vi "Drive Teleop.vi"(9 "POVs":i16[](array[numeric]), 10 "Boolean Array":bool[](array[boolean]), 11 "Axes":dbl[](array[numeric])) -> ()   [LabVIEW 2020]
uses:
  ADIS16470/Typedef/ADIS16470 Status.ctl
  ADIS16470/Typedef/ADIS16470 Data.ctl
  Scaling Types.ctl
  Axes.ctl
  Swerve Mode.ctl
  Buttons.ctl
  <vilib>/Rock Robotics/WPI/Joystick/XBox Buttons Indexer.ctl
  7d80139a-4be2-4268-81d7-0f551d61f1ba.vi
  e6f839d3-980b-4d83-88b4-2e0ae51acaef.vi
  <vilib>/Rock Robotics/Network Tables/NT Write Number.vi
  Drive/Implementation/Infrastructure/Drive Command Helper.vi
panel:
  in  "Rotation Scaling Type":T1
  in  "Translation Scaling Type":T1
  out "ADIS16470 Value":T2
  out "ADIS16470 Status":T3
  in  "Calibrate IMU":bool
  in  "Reset IMU":bool
  in  "Deadband":dbl=0.1
  in  "Disable Rotation":bool
  in  "Disable Y":bool
  in  "Disable X":bool
  in  "omega_max":dbl=180.0
  in  "v_max":dbl=10.0
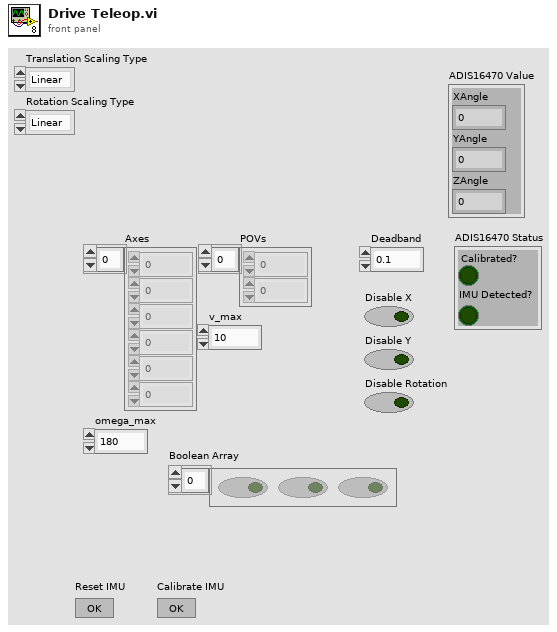
[diagram p1: front panel]
types:
  T1 = typedef "Scaling Types.ctl" = enum16{"Linear", "Square", "Cube", "RSVP5"}
  T2 = typedef "ADIS16470 Data.ctl" = cluster{"XAngle":dbl, "YAngle":dbl, "ZAngle":dbl}
  T3 = typedef "ADIS16470 Status.ctl" = cluster{"Calibrated?":bool, "IMU Detected?":bool}
  T4 = typedef "XBox Buttons Indexer.ctl" = enum16{"A", "B", "X", "Y", "Left Bumper", "Right Bumper", "Back", "Start", "Left Joystick", "Right Joystick"}
  T5 = typedef "Buttons.ctl" = enum16{"A", "B", "X", "Y", "LB", "RB", "menu", "start", "left stick", "right stick"}
  T6 = typedef "Swerve Mode.ctl" = enum16{"Robot Centric", "Field Centric"}
  T7 = typedef "Axes.ctl" = enum16{"LX", "LY", "LT", "RT", "RX", "RY"}
  T8 = typedef "ADIS16470 Device Reference.ctl" = cluster{"DevStatus":errorcluster, "Hardware Config":T9, "Calibration Complete":refnum<notifier>, "Status Reference":refnum<data-value>, "Position Reference":refnum<data-value>, "Velocity Reference":refnum<data-value>, "Sychronous Process VI":T13, "Cmd FIFO":refnum<k33>, "Source":T14, "Data FIFO":refnum<k33>, "Calibration Time (ms)":u32}
  T9 = typedef "ADIS16470 Hardware Configuration.ctl" = cluster{"SPI Clock Rate (Hz)":dbl, "IMU SPI Mode (3)":T10, "IMU Reset Pin":T11, "IMU SPI Bus":T12, "IMU Data Ready Pin":T11, "Stall Config":cluster{"Pow2BytesPerRead":u8, "StallTicks":u16, "CsToSclkTicks":u8}}
  T10 = typedef "WPI_SPIMode.ctl" = enum16{"Mode 0 (Clk Idle Low,Sample on Leading)", "Mode 1 (Clk Idle Low,Sample on Trailing)", "Mode 2 (Clk Idle High,Sample on Leading)", "Mode 3 (Clk Idle High,Sample on Trailing)"}
  T11 = typedef "FPGA_DIOChannel.ctl" = enum8{"DIO 0", "DIO 1", "DIO 2", "DIO 3", "DIO 4", "DIO 5", "DIO 6", "DIO 7", "DIO 8", "DIO 9", "DIO MXP 0", "DIO MXP 1", "DIO MXP 2", "DIO MXP 3", "DIO MXP 4", "DIO MXP 5", "DIO MXP 6", "DIO MXP 7", "DIO MXP 8", "DIO MXP 9", "DIO MXP 10", "DIO MXP 11", "DIO MXP 12", "DIO MXP 13", "DIO MXP 14", "DIO MXP 15", "SPI Port CS1", "SPI Port CS2", "SPI Port CS3", "SPI Port MISO", "SPI Port MOSI", "Invalid"}
  T12 = typedef "spi_bus.ctl" = enum16{"SPI On-Board, CS0", "SPI On-Board, CS1", "SPI On-Board, CS2", "SPI On-Board, CS3", "SPI MXP", "Invalid"}
  T13 = typedef "ADIS16470 Process.ctl" = refnum<vi>
  T14 = typedef "FPGA_CounterEncoderSourceConvertionLVSourceType.ctl" = cluster{"DevStatus":errorcluster, "AnalogTriggerMode?":bool, "DigitalMode":cluster{"DIO Channel":T15}, "AnalogTriggerMode":cluster{"AnalogTriggerIndex":T16, "OutputType":T17}}
  T15 = typedef "FPGA_DIODigitalSourceChannel.ctl" = enum8{"DIO 0", "DIO 1", "DIO 2", "DIO 3", "DIO 4", "DIO 5", "DIO 6", "DIO 7", "DIO 8", "DIO 9", "DIO MXP 0", "DIO MXP 1", "DIO MXP 2", "DIO MXP 3", "DIO MXP 4", "DIO MXP 5", "DIO MXP 6", "DIO MXP 7", "DIO MXP 8", "DIO MXP 9", "DIO MXP 10", "DIO MXP 11", "DIO MXP 12", "DIO MXP 13", "DIO MXP 14", "DIO MXP 15", "SPI Port CS1", "SPI Port CS2", "SPI Port CS3", "SPI Port MISO", "SPI Port MOSI", "Disabled"}
  T16 = typedef "FPGA_AnalogTriggerIndex.ctl" = enum8{"Trig 0", "Trig 1", "Trig 2", "Trig 3", "Trig 4", "Trig 5", "Trig 6", "Trig 7", "Invalid"}
  T17 = typedef "FPGA_AnalogTriggerOutType.ctl" = enum16{"InWindow", "TriggerState", "Rising", "Falling"}
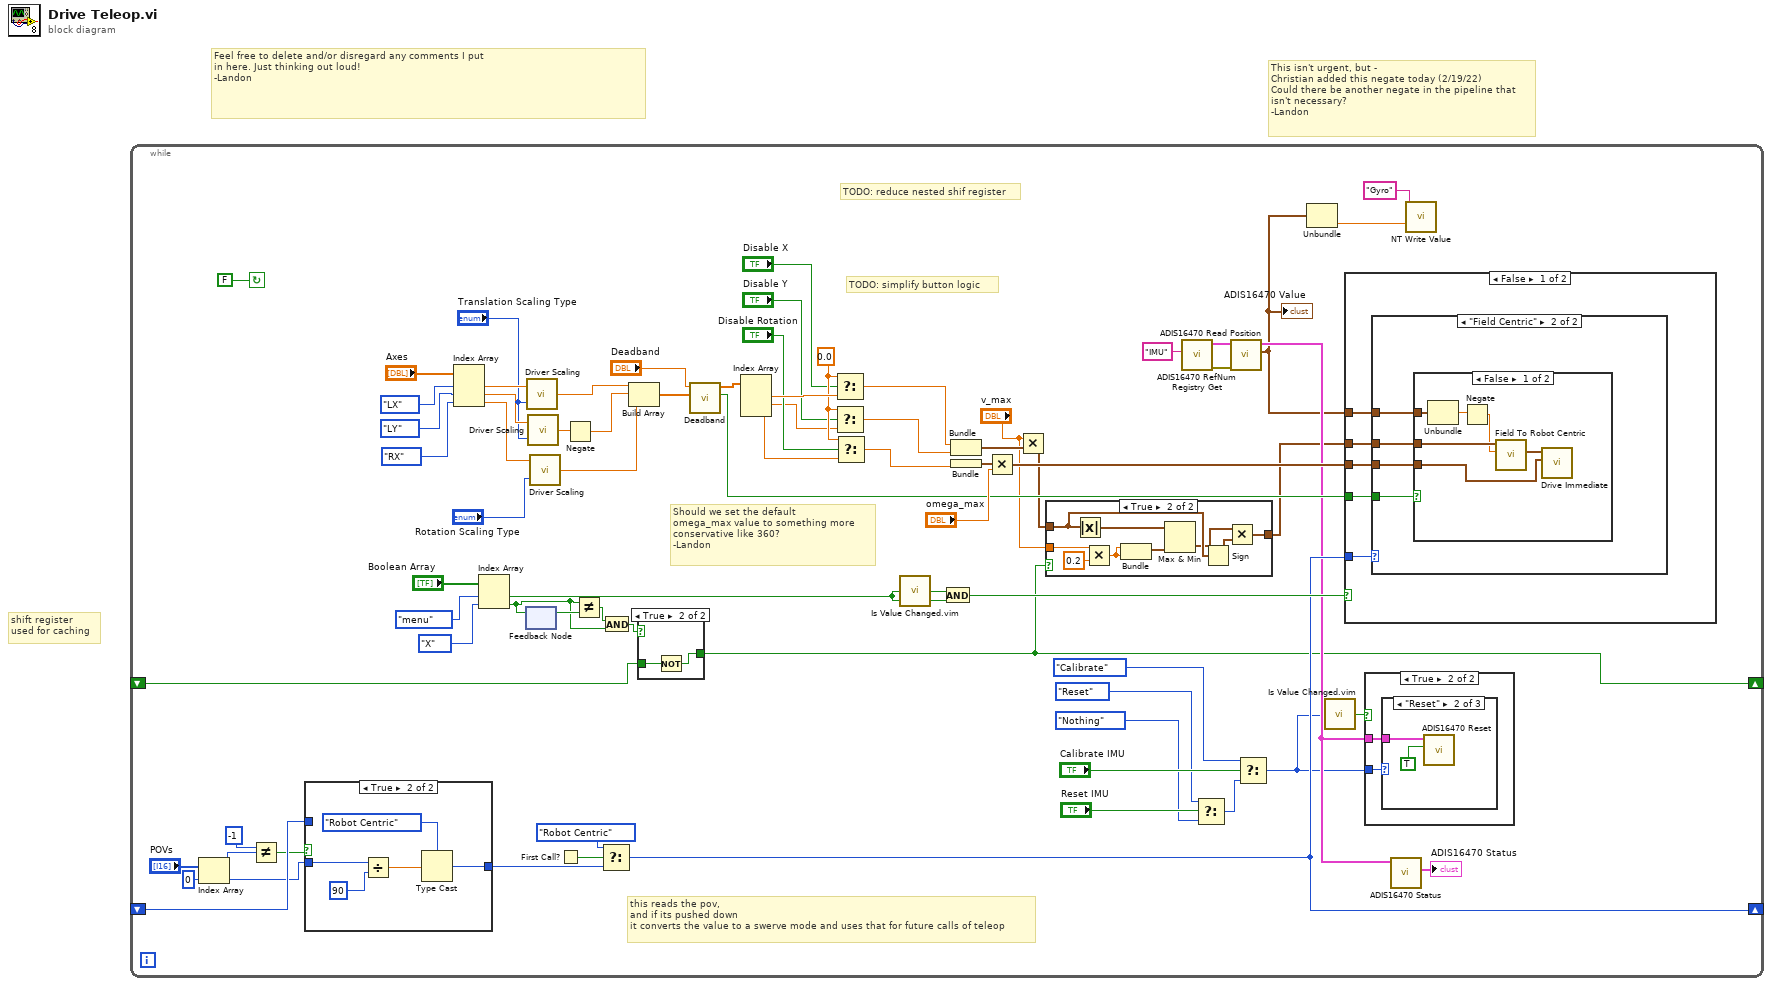
[diagram p0: block diagram]
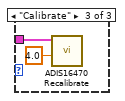
[diagram p6: hidden frame]
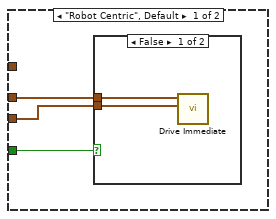
[diagram p7: hidden frame]
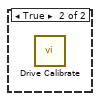
[diagram p10: hidden frame]
diagram:
  # "Feel free to delete and/or disregard any comments I put\nin here. Just thinking out loud!\n-Landon"
  # "This isn't urgent, but -\nChristian added this negate today (2/19/22)\nCould there be another negate in the pipeline that\nisn't necessary?\n-Landon"
  # "shift register\nused for caching"
  n1 = while {
    shift-right: [w39] -> _
    shift-left: _ -> [w65]
    shift-right: [w10] -> _
    shift-left: _ -> [w11]
    stop <- FALSE continue-if-true
    w59 = 0.0 ("f")
    # "Should we set the default\nomega_max value to something more\nconservative like 360?\n-Landon"
    # "TODO: simplify button logic"
    # "TODO: reduce nested shif register"
    # "this reads the pov,\nand if its pushed down\nit converts the value to a swerve mode and uses that for future calls of teleop"
    n2 = Index Array(array="POVs", index=0) -> (element=w46:i16)
    n3 = Not Equal?(x=-1, y=w46) -> (x != y?=w47:bool)
    n4 = case shown="True" w47 {
      tunnel: w46 -> [_ w118]
      tunnel: [w113 w114] -> w66
      tunnel: w65 -> [w113 _]
      frame False {
      }
      frame True {
        n5 = Divide(x=w118, y=90) -> (x/y=w115:dbl)
        n6 = Type Cast(type=Swerve_Mode."Robot Centric" ("Swerve Mode"), x=w115) -> (*(type *) &x=w114:T6)
      }
    }
    n7 = Index Array(array="Axes", index #1=Axes."LX" ("Axes"), index #2=Axes."LY" ("Axes"), index #3=Axes."RX" ("Axes")) -> (element #1=w24:dbl, element #2=w23:dbl, element #3=w22:dbl)
    n8 = Index Array(array="Boolean Array", index #1=Buttons."menu" ("Button"), index #2=XBox_Buttons_Indexer."X" ("XBox Buttons")) -> (element #1=w13:bool, element #2=w5:bool)
    n9 = feedback-in #1(w5) -> ()
    n10 = feedback #1() -> (w12:bool)  [unwired: 1 in]
    n11 = call "Driver Scaling.vi"("Scaling Type"="Translation Scaling Type", "x"=w24) -> ("y"=w17:dbl)
    n12 = call "Driver Scaling.vi"("Scaling Type"="Translation Scaling Type", "x"=w23) -> ("y"=w19:dbl)
    n13 = call "Driver Scaling.vi"("Scaling Type"="Rotation Scaling Type", "x"=w22) -> ("y"=w16:dbl)
    n14 = First Call?() -> (First Call?: T/F=w68:bool)
    n15 = Negate(x=w19) -> (-x=w18:dbl)
    n16 = Not Equal?(x=w5, y=w12) -> (x != y?=w6:bool)
    n17 = Select(t=Swerve_Mode."Robot Centric" ("Swerve Mode"), s=w68, f=w66) -> (s? t:f=w39:T6)
    n18 = And(x=w6, y=w5) -> (x .and. y?=w4:bool)
    n19 = Build Array(w17, w18, w16) -> (w15:dbl[])
    n20 = case shown="True" w4 {
      tunnel: w11 -> [w84 w86]
      tunnel: [w84 w85] -> w10
      frame False {
      }
      frame True {
        n21 = Not(x=w86) -> (.not. x?=w85:bool)
      }
    }
    n22 = call "Deadband.vi"("Inputs"=w15, "Deadband"="Deadband") -> ("Is Zero?"=w40:bool, "Ouptuts"=w41:dbl[])  [unwired: 8 in]
    n23 = Index Array(array=w41) -> (element #1=w61:dbl, element #2=w51:dbl, element #3=w60:dbl)  [unwired: 3 in]
    n24 = Select(t=w59, s="Disable X", f=w61) -> (s? t:f=w55:dbl)
    n25 = Select(t=w59, s="Disable Y", f=w51) -> (s? t:f=w54:dbl)
    n26 = Select(t=w59, s="Disable Rotation", f=w60) -> (s? t:f=w53:dbl)
    n27 = call "Is Value Changed.vim"("value"=w13) -> ("changed or first call?"=w43:bool)
    n28 = And(x=w43, y=w13) -> (x .and. y?=w45:bool)
    n29 = Bundle("upper limit"=w55, "upper limit"=w54) -> (w52:cluster{"upper limit":dbl, "upper limit":dbl})  [unwired: 1 in]
    n30 = Bundle("upper limit"=w53) -> (w64:cluster{"upper limit":dbl})  [unwired: 1 in]
    n31 = Multiply(x=w64, y="omega_max") -> (x*y=w62:cluster{"upper limit":dbl})
    n32 = Multiply(x="v_max", y=w52) -> (x*y=w9:cluster{"upper limit":dbl, "upper limit":dbl})
    n33 = case shown="True" w10 {
      tunnel: w9 -> [w74 w78]
      tunnel: "v_max" -> [_ w81]
      tunnel: [w74 w76] -> w7
      frame False {
      }
      frame True {
        n34 = Absolute Value(x=w78) -> (abs(x)=w83:cluster{"upper limit":dbl, "upper limit":dbl})
        n35 = Multiply(x=w81, y=0.2) -> (x*y=w79:dbl)
        n36 = Bundle(w79, w79) -> (w82:cluster{dbl, dbl})  [unwired: 1 in]
        n37 = Max & Min(x=w83, y=w82) -> (min(x,y)=w75:cluster{dbl, dbl})  [unwired: 1 out]
        n38 = Sign(1:w78) -> (0:w77:cluster{"upper limit":dbl, "upper limit":dbl})
        n39 = Multiply(x=w75, y=w77) -> (x*y=w76:cluster{dbl, dbl})
      }
    }
    n40 = call "ADIS16470 RefNum Registry Get.vi"("refnum name"="IMU") -> ("error out"=w38:errorcluster, "ADIS16470DevRef out"=w37:T8)  [unwired: 9 in]
    n41 = Select(t=enum16{"Nothing", "Calibrate", "Reset"}."Reset", s="Reset IMU", f=enum16{"Nothing", "Calibrate", "Reset"}."Nothing") -> (s? t:f=w31:enum16{"Nothing", "Calibrate", "Reset"})
    n42 = call "ADIS16470 Read Position.vi"("error in (no error)"=w38, "ADIS16470DevRef"=w37) -> ("ADIS16470 Value"=w3:T2, "ADIS16470DevRef"=w30:T8)  [unwired: 6 in, 2 out]
    "ADIS16470 Value" <- w3
    n43 = Select(t=enum16{"Nothing", "Calibrate", "Reset"}."Calibrate", s="Calibrate IMU", f=w31) -> (s? t:f=w28:enum16{"Nothing", "Calibrate", "Reset"})
    n44 = Unbundle(w3) -> ("ZAngle"=w1:dbl)  [unwired: 2 out]
    n45 = call "Is Value Changed.vim"("value"=w28) -> ("changed or first call?"=w27:bool)
    n46 = case shown="False" w45 {
      tunnel: w62 -> [w97 _]
      tunnel: w7 -> [w96 _]
      tunnel: w40 -> [w95 _]
      tunnel: w39 -> [w94 _]
      tunnel: w3 -> [w93 _]
      frame False {
        n47 = case shown="\"Field Centric\"" w94 {
          tunnel: w97 -> [w100 w105]
          tunnel: w96 -> [w99 w106]
          tunnel: w95 -> [w98 w103]
          tunnel: w93 -> [_ w104]
          frame "Robot Centric", Default {
            n48 = case shown="False" w98 {
              tunnel: w100 -> [w101 _]
              tunnel: w99 -> [w102 _]
              frame False {
                n49 = call "Drive Immediate.vi"("Rotational"=w101, "Translational"=w102) -> ()  [unwired: 9 in, 1 out]
              }
              frame True {
              }
            }
          }
          frame "Field Centric" {
            n50 = case shown="False" w103 {
              tunnel: w106 -> [w112 _]
              tunnel: w105 -> [w110 _]
              tunnel: w104 -> [w109 _]
              frame False {
                n51 = Unbundle(w109) -> ("YAngle"=w108:dbl)  [unwired: 2 out]
                n52 = Negate(x=w108) -> (-x=w107:dbl)
                n53 = call "Field To Robot Centric.vi"("IMU Value (offset)"=w107, "Translation Joystick"=w112) -> ("Robot Centric Vector"=w111:cluster{dbl, dbl})  [unwired: 8 in, 1 out]
                n54 = call "Drive Immediate.vi"("Rotational"=w110, "Translational"=w111) -> ()  [unwired: 9 in, 1 out]
              }
              frame True {
              }
            }
          }
        }
      }
      frame True {
        n55 = call "Drive Calibrate.vi"() -> ()  [unwired: 11 in, 1 out]
      }
    }
    n56 = case shown="True" w27 {
      tunnel: w28 -> [_ w88]
      tunnel: w30 -> [_ w87]
      frame False {
      }
      frame True {
        n57 = case shown="\"Reset\"" w88 {
          tunnel: w87 -> [_ w90 w92]
          frame "Nothing", Default {
          }
          frame "Reset" {
            n58 = call "ADIS16470 Reset.vi"("Reset? (T)"=TRUE, "ADIS16470DevRef"=w90) -> ()  [unwired: 8 in, 2 out]
          }
          frame "Calibrate" {
            n59 = call "ADIS16470 Recalibrate.vi"("Calibration Time (4s)"=4.0, "ADIS16470DevRef in"=w92) -> ()  [unwired: 8 in, 2 out]
          }
        }
      }
    }
    n60 = call "ADIS16470 Status.vi"("ADIS16470DevRef"=w30) -> ("ADIS16470 Status"=→"ADIS16470 Status":T3)  [unwired: 8 in, 2 out]
    n61 = call-poly <vilib>:"NT Write Value.vi"("Numeric"=w1, "Name"="Gyro") -> ()  [unwired: 9 in, 1 out]
  }
